vi "NanotecSMCPDDriver.set number of steps.vi"(0 "VISA resource name":refnum<visa-resource-name>, 1 "contollerID":i32=-1, 3 "nOfSteps [uSteps]":i32, 5 "error in (no error)":errorcluster) -> (14 "VISA resource name out":refnum<visa-resource-name>, 15 "contollerID out":i32=-1, 19 "error out":errorcluster)   [LabVIEW 2015, in "NanotecSMCPDDriver.lvlib"]
doc: "Sets the number of steps that will be used for the next movement."
uses:
  NanotecSMCPDDriver.lvlib
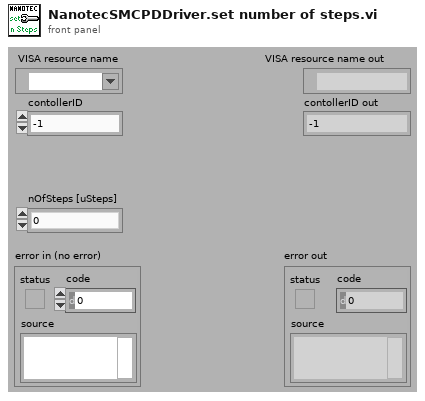
[diagram p1: front panel]
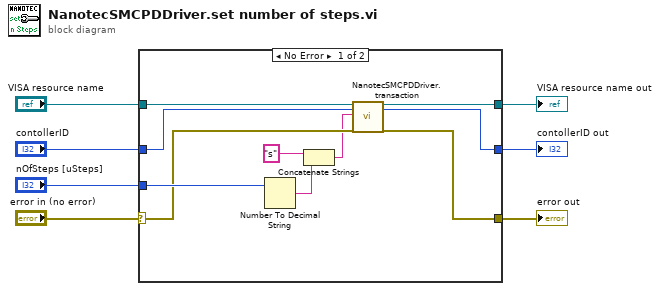
[diagram p0: block diagram]
diagram:
  n1 = case shown="No Error" "error in (no error)" {
    selector: "error in (no error)" -> [w11 w18]
    tunnel: [w16 w20] -> w7
    tunnel: [w15 w18] -> w6
    tunnel: "VISA resource name" -> [w13 w20]
    tunnel: "contollerID" -> [w12 w19]
    tunnel: [w17 w19] -> w3
    tunnel: "nOfSteps [uSteps]" -> [w14 _]
    frame No Error {
      n2 = Number To Decimal String(number=w14) -> (decimal integer string=w10:string)  [unwired: 1 in]
      n3 = Concatenate Strings("s" ("commandString"), w10) -> (w8:string)
      n4 = call "NanotecSMCPDDriver.transaction.vi"("VISAresource"=w13, "contollerID"=w12, "commandString"=w8, "error in (no error)"=w11) -> ("VISAresource out"=w16:refnum<visa-resource-name>, "contollerID out"=w17:i32, "error out"=w15:errorcluster)  [unwired: 10 in, 3 out]
    }
    frame Error {
    }
  }
  "VISA resource name out" <- w7
  "error out" <- w6
  "contollerID out" <- w3
